vi "checkoffMission.vi"(8 "error in (no error)":errorcluster, 11 "GenericMission in":refnum<class "GenericMission.lvclass">) -> (0 "error out":errorcluster, 3 "GenericMission out":refnum<class "GenericMission.lvclass">)   [LabVIEW 2013, in "GenericMission.lvclass"]
doc: "check off mission (set done? to TRUE)"
uses:
  GenericMission.lvclass
  GenericMission.lvclass/GenericMission.ctl
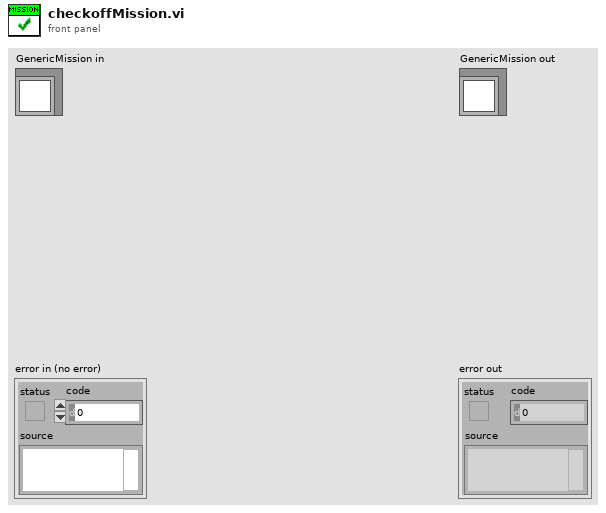
[diagram p1: front panel]
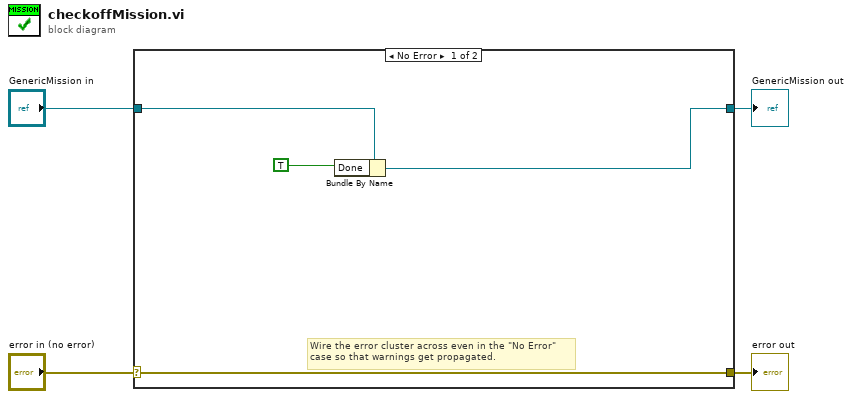
[diagram p0: block diagram]
diagram:
  n1 = case shown="No Error" "error in (no error)" {
    selector: "error in (no error)" -> [w8 w10]
    tunnel: [w8 w10] -> w3
    tunnel: [w5 w9] -> w1
    tunnel: "GenericMission in" -> [w6 w9]
    frame No Error {
      # "Wire the error cluster across even in the \"No Error\"\ncase so that warnings get propagated."
      n2 = Bundle By Name(cluster=w6, "Done"=TRUE) -> (w5:refnum<class "GenericMission.lvclass">)
    }
    frame Error {
    }
  }
  "error out" <- w3
  "GenericMission out" <- w1
